vi "tmp make sample arr.vi"(6 "Bindata & descr in":T1, 7 "type":dbl, 8 "error in (no error)":errorcluster, 9 "dims":u8=3 min=1 max=3, 11 "kwarg_name":string="testarg") -> (0 "error out":errorcluster, 1 "Array 3D":dbl[][][](array[numeric]) format="%.2f", 2 "Array 2D":dbl[][](array[numeric]) format="%.2f", 3 "Array 1D":dbl[](array[numeric]) format="%.2f", 4 "Bindata & descr out":T1)   [LabVIEW 2018]
uses:
  Bindata&description.ctl
  Bindata description.ctl
  f894a9dc-d91c-43e8-b7ce-34de6020b674.vi
  220964fc-f472-4a25-bc8a-83b984c513e6.vi
  b0e3a4eb-cc81-4f43-a5e1-c85d6dd74692.vi
  220964fc-f472-4a25-bc8a-83b984c513e6.vi/ff0151bc-c526-4cc1-912e-66cba6b8abc3.vi
  b0e3a4eb-cc81-4f43-a5e1-c85d6dd74692.vi/a5afbe4f-d4b1-449a-9f40-01c9ed494de2.vi
  220964fc-f472-4a25-bc8a-83b984c513e6.vi/ff0151bc-c526-4cc1-912e-66cba6b8abc3.vi/b4d3508f-4117-4ac7-910d-1a9cb65e6960.vi
  b0e3a4eb-cc81-4f43-a5e1-c85d6dd74692.vi/a5afbe4f-d4b1-449a-9f40-01c9ed494de2.vi/85ed65b8-73e1-4959-8d99-4904b7525b09.vi
  220964fc-f472-4a25-bc8a-83b984c513e6.vi/ff0151bc-c526-4cc1-912e-66cba6b8abc3.vi/b4d3508f-4117-4ac7-910d-1a9cb65e6960.vi/a513af8e-c39d-4c9e-a0c5-0ef488f5c59e.vi
  b0e3a4eb-cc81-4f43-a5e1-c85d6dd74692.vi/a5afbe4f-d4b1-449a-9f40-01c9ed494de2.vi/85ed65b8-73e1-4959-8d99-4904b7525b09.vi/326e0331-4022-4a24-9bc6-2447645c43c9.vi
  check ID validity.vi
  LV-Julia_ZMQ-Roundtrip_lib.lvlib
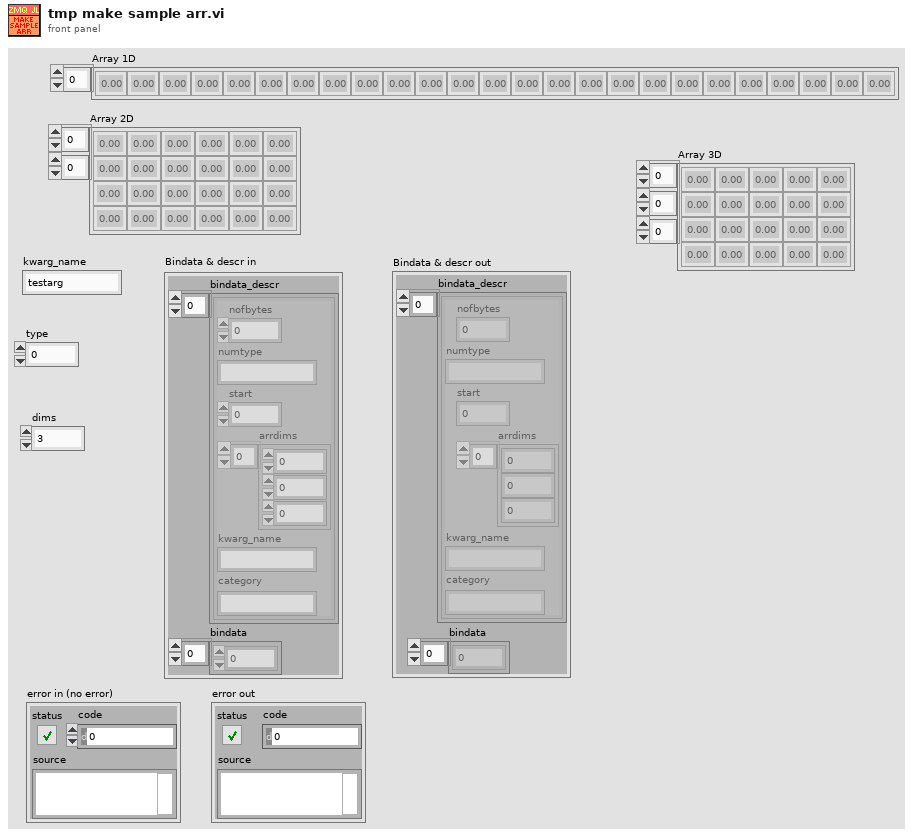
[diagram p1: front panel]
types:
  T1 = typedef "Bindata&description.ctl" = cluster{"bindata_descr":T2[], "bindata":u8[]}
  T2 = typedef "LV-Julia_ZMQ-Roundtrip_lib.lvlib/Bindata description.ctl" = cluster{"nofbytes":i32, "numtype":string, "start":i32, "arrdims":i32[], "kwarg_name":string, "category":string}
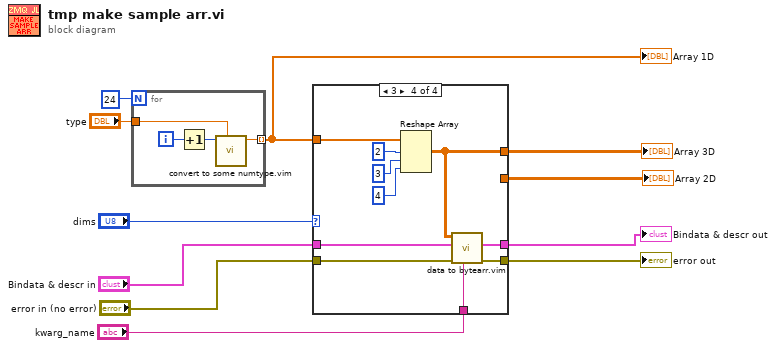
[diagram p0: block diagram]
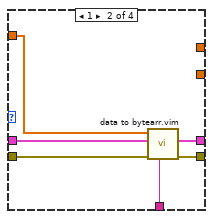
[diagram p3: hidden frame]
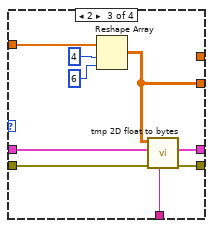
[diagram p4: hidden frame]
diagram:
  n1 = for {
    N: 24 -> [_]
    tunnel: [w13] -> w10 mode=indexing
    tunnel: "type" -> [w12]
    i -> [w15]
    n2 = Increment(x=w15) -> (x+1=w14:i32)
    n3 = call "convert to some numtype.vim"("type"=w12, "Numeric in"=w14) -> ("Numeric out"=w13:dbl)  [unwired: 9 in]
  }
  "Array 1D" <- w10
  n4 = case shown="3" "dims" {
    tunnel: [_ _ _ w41] -> w11
    tunnel: w10 -> [_ w22 w29 w37]
    tunnel: "kwarg_name" -> [_ w21 w28 w36]
    tunnel: "error in (no error)" -> [w16 w20 w27 w35]
    tunnel: [w16 w19 w26 w34] -> w4
    tunnel: [_ w18 w25 w33] -> w3
    tunnel: [_ _ w24 _] -> w2
    tunnel: "Bindata & descr in" -> [_ w17 w23 w32]
    frame 0, Default {
    }
    frame 1 {
      n5 = call "data to bytearr.vim"("kwarg_name"=w21, "error in (no error)"=w20, "Bindata & descr in"=w17, "data in"=w22) -> ("error out"=w19:errorcluster, "Bindata & descr out"=w18:T1)  [unwired: 5 in, 1 out]
    }
    frame 2 {
      n6 = Reshape Array(w29, 4 ("dimension size"), 6 ("dimension size")) -> (w24:dbl[][])
      n7 = call "tmp 2D float to bytes.vi"("kwarg_name"=w28, "error in (no error)"=w27, "Bindata & descr in"=w23, "data in"=w24) -> ("error out"=w26:errorcluster, "Bindata & descr out"=w25:T1)  [unwired: 5 in, 1 out]
    }
    frame 3 {
      n8 = Reshape Array(w37, 2 ("dimension size"), 3 ("dimension size"), 4 ("dimension size")) -> (w41:dbl[][][])
      n9 = call "data to bytearr.vim"("kwarg_name"=w36, "error in (no error)"=w35, "Bindata & descr in"=w32, "data in"=w41) -> ("error out"=w34:errorcluster, "Bindata & descr out"=w33:T1)  [unwired: 5 in, 1 out]
    }
  }
  "Array 3D" <- w11
  "Bindata & descr out" <- w3
  "error out" <- w4
  "Array 2D" <- w2
